vi "setZero.vi"(7 "Motor":i32, 8 "error in (no error)":errorcluster, 9 "Device Address In":i32, 10 "DeviceKey In":string, 11 "CmdLib In":refnum<k24>) -> (0 "error out":errorcluster, 1 "Device Address Out":i32, 2 "DeviceKey Out":string, 3 "CmdLib Out":refnum<k24>)   [LabVIEW 2018]
uses:
  Device VIs/CmdLib.dll
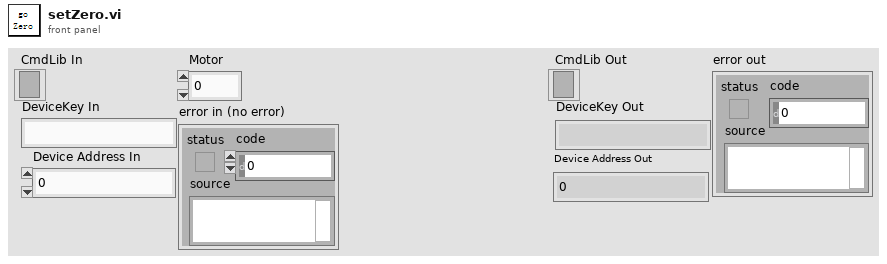
[diagram p1: front panel]
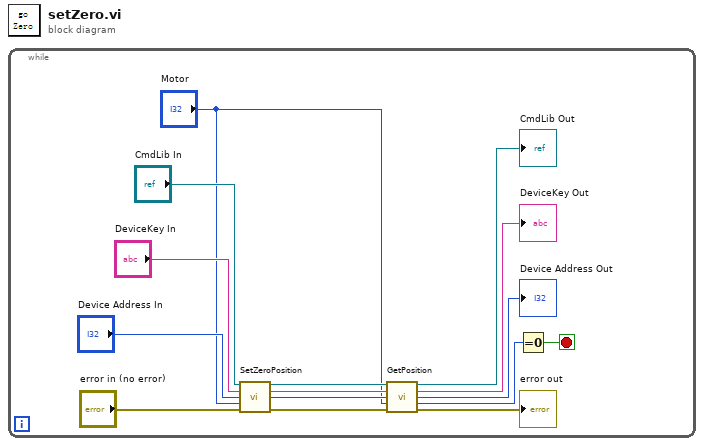
[diagram p0: block diagram]
diagram:
  n1 = while {
    stop <- w1 stop-if-true
    n2 = call "SetZeroPosition.vi"("CmdLib In"="CmdLib In", "DeviceKey In"="DeviceKey In", "Device Address In"="Device Address In", "Motor"="Motor", "error in (no error)"="error in (no error)") -> ("CmdLib Out"=w15:refnum<k24>, "DeviceKey Out"=w14:string, "Device Address Out"=w13:i32, "error out"=w8:errorcluster)  [unwired: 7 in]
    n3 = call "GetPosition.vi"("CmdLib In"=w15, "DeviceKey In"=w14, "Device Address In"=w13, "Motor"="Motor", "error in (no error)"=w8) -> ("CmdLib Out"=→"CmdLib Out":refnum<k24>, "DeviceKey Out"=→"DeviceKey Out":string, "Device Address Out"=→"Device Address Out":i32, "Position"=w2:i32, "error out"=→"error out":errorcluster)  [unwired: 6 in]
    n4 = Equal To 0?(x=w2) -> (x = 0?=w1:bool)
  }
